vi "(5-23-2024) Read Barcode From Cognex Scanner.vi"() -> ()   [LabVIEW 2020]
doc: "This VI opens a connection to a Cognex DM200 scanner, initiate a read request and wait for the read data string or a timeout."
panel:
  in  "Timeout ms":i32
  out "Time Out":bool
  out "Raw Data Read":string
  in  "IP Address Barcode Reader":string="192.168.1.173"
  # "Overview: Demonstrates how to read a barcode from a Cognex scanner. \n\nInstructions: \n1. Set the IP Address and the Timout for the scanner.\n2. Run the VI."
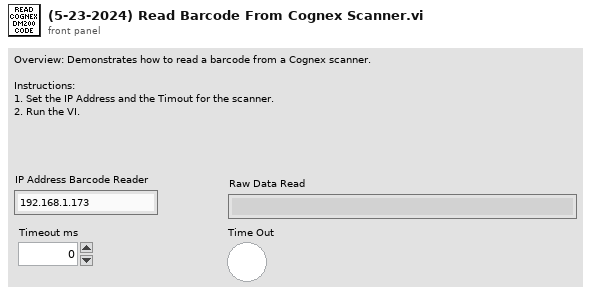
[diagram p1: front panel]
types:
  T1 = enum16{"Standard", "Buffered", "CRLF", "Immediate"}
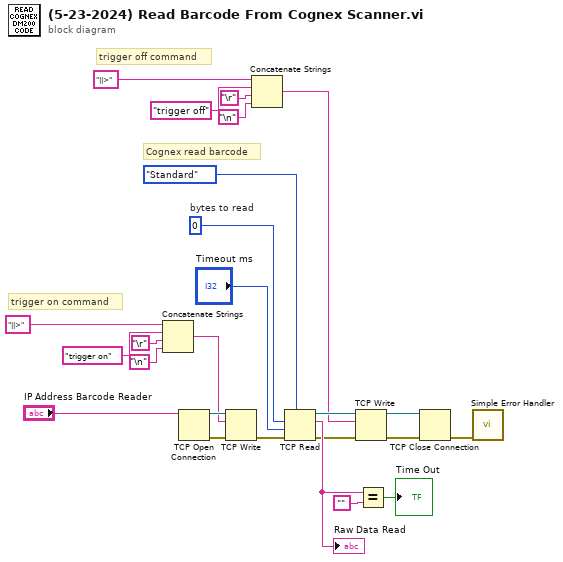
[diagram p0: block diagram]
diagram:
  w11 = 0  # bytes to read
  # "Cognex read barcode"
  # "trigger off command"
  # "trigger on command"
  n1 = Concatenate Strings("||>" ("string"), "trigger on" ("string"), "\r", "\n") -> (w13:string)
  n2 = TCP Open Connection(address="IP Address Barcode Reader") -> (connection ID=w15:refnum<k5>, error out=w14:errorcluster)  [unwired: 4 in]
  n3 = TCP Write(connection ID=w15, data in=w13, error in (no error)=w14) -> (error out=w12:errorcluster)  [unwired: 1 in, 2 out]
  n4 = Concatenate Strings("||>" ("string"), "trigger off" ("string"), "\r", "\n") -> (w7:string)
  n5 = TCP Read(bytes to read=w11, error in (no error)=w12, 7:T1."Standard" ("mode (standard)"), 9:"Timeout ms") -> (connection ID out=w9:refnum<k5>, data out=w10:string, error out=w6:errorcluster)  [unwired: 1 in]
  "Raw Data Read" <- w10
  n6 = TCP Write(connection ID=w9, data in=w7, error in (no error)=w6) -> (connection ID out=w8:refnum<k5>, error out=w5:errorcluster)  [unwired: 1 in, 1 out]
  n7 = Equal?(x=w10, y="") -> (x = y?=→"Time Out":bool)
  n8 = TCP Close Connection(connection ID=w8, error in (no error)=w5) -> (error out=w4:errorcluster)  [unwired: 1 in, 1 out]
  n9 = call <vilib>:"Simple Error Handler.vi"("error in (no error)"=w4) -> ()  [unwired: 4 in, 5 out]
